vi "Configure Channel Enable.vi"(8 "error in (no error)":errorcluster, 9 "Enable Channel (T: Enable)":bool=TRUE, 10 "Channel Select":enum16{"Channel 1", "Channel 2", "Channel 3"}(ring), 11 "Visa Resource Name IN":refnum<visa-resource-name>) -> (0 "error out":errorcluster, 3 "Visa Resource Name OUT":refnum<visa-resource-name>)   [LabVIEW 2018, in "Keithley KE22xx Series.lvlib"]
doc: "To Enable/Disable a specified channel. \n\nNote: Once any channel is disabled, it is not possible to make output power state on for that channel untill the same channel has been enabled."
uses:
  Keithley KE22xx Series.lvlib
panel:
  # "© 2012 Keithley Instruments, Inc. ALL RIGHTS RESERVED"
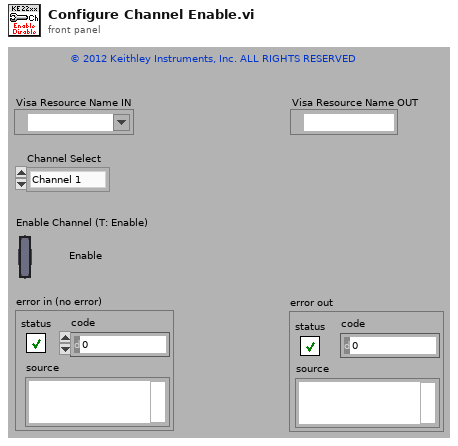
[diagram p1: front panel]
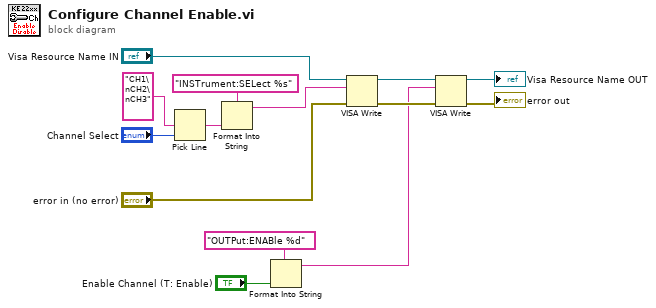
[diagram p0: block diagram]
diagram:
  n1 = Pick Line(multi-line string="CH1\nCH2\nCH3", line index="Channel Select") -> (output string=w6:string)  [unwired: 1 in]
  n2 = Format Into String(format string="INSTrument:SELect %s", w6) -> (resulting string=w4:string)  [unwired: 2 in, 1 out]
  n3 = Format Into String(format string="OUTPut:ENABle %d", "Enable Channel (T: Enable)") -> (resulting string=w2:string)  [unwired: 2 in, 1 out]
  n4 = VISA Write(VISA resource name="Visa Resource Name IN", write buffer=w4, error in (no error)="error in (no error)") -> (VISA resource name out=w11:refnum<visa-resource-name>, error out=w10:errorcluster)  [unwired: 1 out]
  n5 = VISA Write(VISA resource name=w11, write buffer=w2, error in (no error)=w10) -> (VISA resource name out=→"Visa Resource Name OUT":refnum<visa-resource-name>, error out=→"error out":errorcluster)  [unwired: 1 out]
